vi "FFT Power Spectrum and PSD for N Chan.vi"(4 "window parameter":dbl=nan, 5 "export mode":T1 items=["Power Spectrum", "Power Spectral Density"], 6 "averaging parameters":T3={"averaging mode"=enum."No averaging", "weighting mode"=enum."Exponential", "number of averages"=10} {"number of averages" min=1}, 7 "restart averaging (F)":bool, 8 "error in (no error)":errorcluster, 9 "dB On (F)":bool, 10 "window":T2=1 items=["Rectangle"=0, "Hanning"=1, "Hamming"=2, "Blackman-Harris"=3, "Exact Blackman"=4, "Blackman"=5, "Flat Top"=6, "4 Term B-Harris "=7, "7 Term B-Harris"=8, "Low Sidelobe"=9, "Blackman Nuttall"=11, "Triangle"=30, "Bartlett-Hanning"=31, "Bohman"=32, "Parzen"=33, "Welch"=34, "Kaiser"=60, "Dolph-Chebyshev"=61, "Gaussian"=62], 11 "time signals":waveform(dbl)[](array[waveform])) -> (0 "error out":errorcluster, 1 "averages completed":dbl, 2 "averaging done":bool, 3 "Power Spectrum / PSD":cluster{"f0":dbl, "df":dbl, "magnitude":dbl[]}[](array[cluster]) {"magnitude" format="%.2p"; "f0" format="%.2p"; "df" format="%.2p"})   [LabVIEW 2020, in "NI_MAPro.lvlib"]
doc: "Computes the averaged auto power spectrum of <B>time signal</B>. Wire data to the <B>time signal</B> input to determine the polymorphic instance to use or manually select the instance."
uses:
  NI_MAPro.lvlib
  windowTd.ctl
  Power Spectrum and PSD Export Mode.ctl
  NI_AALPro.lvlib
  NI_MABase.lvlib
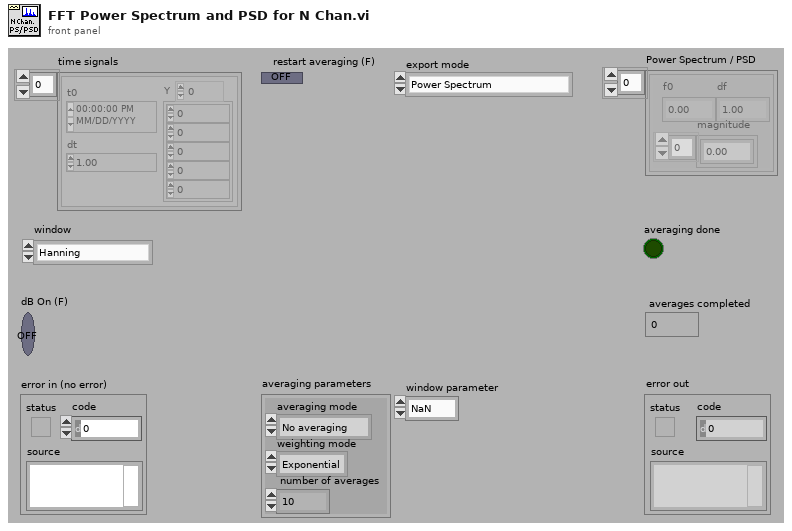
[diagram p1: front panel]
types:
  T1 = typedef "NI_MAPro.lvlib/Power Spectrum and PSD Export Mode.ctl" = u16
  T2 = typedef "NI_AALPro.lvlib/windowTd.ctl" = u32
  T3 = cluster{"averaging mode":enum16{"No averaging", "Vector averaging", "RMS averaging", "Peak hold"}, "weighting mode":enum16{"Linear", "Exponential"}, "number of averages":u32}
  T4 = cluster{"block size":i32, "dt":dbl, "spectrum parameters":cluster{"averaging parameters":cluster{"averaging mode":enum16{"No averaging", "Vector averaging", "RMS averaging", "Peak hold"}, "weighting mode":enum16{"Linear", "Exponential"}, "number of averages":u32}, "window":T2}, "df":dbl, "averages completed":dbl, "complex spectrum":cdb[], "real spectrum":dbl[], "t0 history":dbl, "dt history":dbl, "timestamp":dbl, "lin avg done":bool}
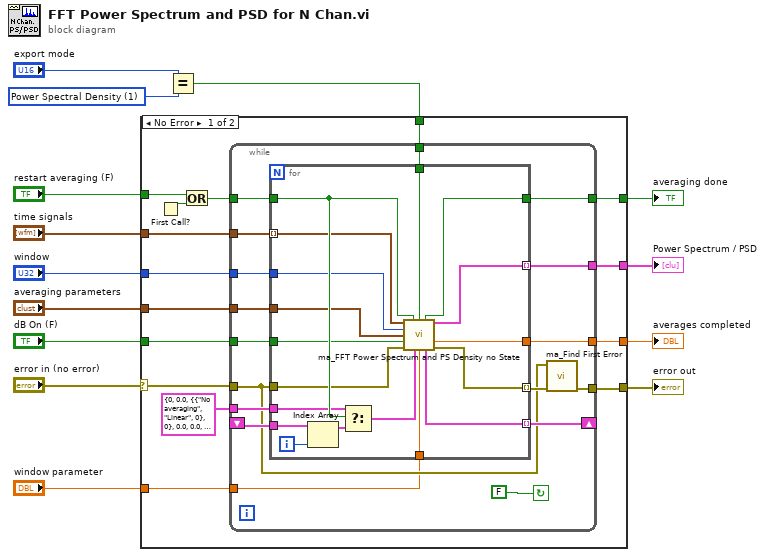
[diagram p0: block diagram]
diagram:
  w3 = T1 1 items=["Power Spectrum", "Power Spectral Density"] ("export mode 2")
  n1 = Equal?(x="export mode", y=w3) -> (x = y?=w2:bool)
  n2 = case shown="No Error" "error in (no error)" {
    selector: "error in (no error)" -> [w26 w65]
    tunnel: [w27 w65] -> w13
    tunnel: "restart averaging (F)" -> [w24 _]
    tunnel: "time signals" -> [w23 _]
    tunnel: "window" -> [w22 _]
    tunnel: "averaging parameters" -> [w21 _]
    tunnel: "dB On (F)" -> [w20 _]
    tunnel: [w19 _] -> w7
    tunnel: [w18 _] -> w6
    tunnel: [w17 _] -> w5
    tunnel: w2 -> [w16 _]
    tunnel: "window parameter" -> [w15 _]
    frame No Error {
      n3 = First Call?() -> (First Call?: T/F=w29:bool)
      n4 = Or(x=w24, y=w29) -> (x .or. y?=w28:bool)
      n5 = while {
        tunnel: w22 -> [w38]
        tunnel: w26 -> [w32]
        tunnel: w23 -> [w37]
        tunnel: w21 -> [w36]
        tunnel: w28 -> [w42]
        tunnel: [w46] -> w19
        tunnel: [w45] -> w17
        tunnel: [w44] -> w18
        shift-right: [w43] -> _
        shift-left: _ -> [w41]
        tunnel: T4 {"block size"=0, "dt"=0.0, "spectrum parameters"={"averaging parameters"={"averaging mode"=enum."No averaging", "weighting mode"=enum."Linear", "number of averages"=0}, "window"=0}, "df"=0.0, "averages completed"=0.0, "complex spectrum"=[], "real spectrum"=[], "t0 history"=0.0, "dt history"=0.0, "timestamp"=0.0, "lin avg done"=FALSE} ("state info") -> [w40]
        tunnel: w20 -> [w39]
        tunnel: [w33] -> w27
        tunnel: w16 -> [w31]
        tunnel: w15 -> [w30]
        stop <- FALSE continue-if-true
        n6 = for {
          tunnel: [w64] -> w46
          tunnel: [w63] -> w45
          tunnel: [w62] -> w44 mode=indexing
          tunnel: [w61] -> w34 mode=indexing
          tunnel: [w60] -> w43 mode=indexing
          tunnel: w42 -> [w59]
          tunnel: w41 -> [w51]
          tunnel: w40 -> [w57]
          tunnel: w32 -> [w56]
          tunnel: w39 -> [w55]
          tunnel: w38 -> [w54]
          tunnel: w37 -> [w53] mode=indexing
          tunnel: w36 -> [w52]
          tunnel: w31 -> [w48]
          tunnel: w30 -> [w47]
          i -> [w50]
          n7 = Index Array(array=w51, index=w50) -> (element=w49:T4)
          n8 = Select(t=w57, s=w59, f=w49) -> (s? t:f=w58:T4)
          n9 = call "ma_FFT Power Spectrum and PS Density no State.vi"("time signal"=w53, "restart averaging (F)"=w59, "ps density"=w48, "window"=w54, "averaging parameters"=w52, "dB On (F)"=w55, "error in"=w56, "state info"=w58, "window parameter"=w47) -> ("averaging done"=w64:bool, "power spectrum"=w62:cluster{"f0":dbl, "df":dbl, "magnitude":dbl[]}, "averages completed"=w63:dbl, "state info"=w60:T4, "error out"=w61:errorcluster)  [unwired: 2 out]
        }
        n10 = call "ma_Find First Error.vi"("error array in"=w34, "error in 1 (no error)"=w32) -> ("error out"=w33:errorcluster)  [unwired: 2 in, 3 out]
      }
    }
    frame Error {
    }
  }
  "error out" <- w13
  "averages completed" <- w5
  "averaging done" <- w7
  "Power Spectrum / PSD" <- w6
